vi "addition.vi"() -> ()   [LabVIEW 2020]
panel:
  out "Sum":dbl
  in  "Num2":dbl
  in  "Number1":dbl
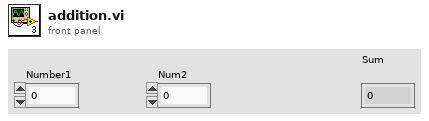
[diagram p1: front panel]
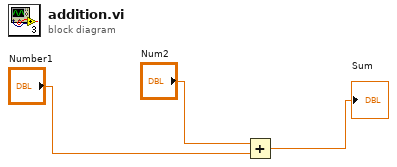
[diagram p0: block diagram]
diagram:
  n1 = Add(x="Num2", y="Number1") -> (x+y=→"Sum":dbl)
